vi "Add Menu Items.vi"(7 "Menu control":enum16{"Pulse", "Post-process", "Monitor"}(ring), 8 "error in (no error)":errorcluster, 9 "Reset":bool, 10 "Item Names":string[](array[string]), 11 "Monitor-Pulse in":refnum<class "Monitor-Pulse.lvclass">) -> (0 "error out":errorcluster, 3 "Monitor-Pulse out":refnum<class "Monitor-Pulse.lvclass">)   [LabVIEW 2016, in "Monitor-Pulse.lvclass"]
uses:
  Monitor-Pulse.lvclass
  Monitor-Pulse.lvclass/Monitor-Pulse.ctl
  Controllers/Application Controller/Application Controller.lvclass
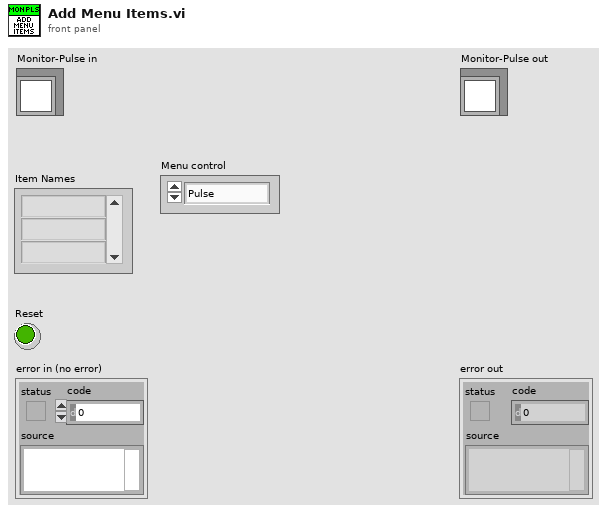
[diagram p1: front panel]
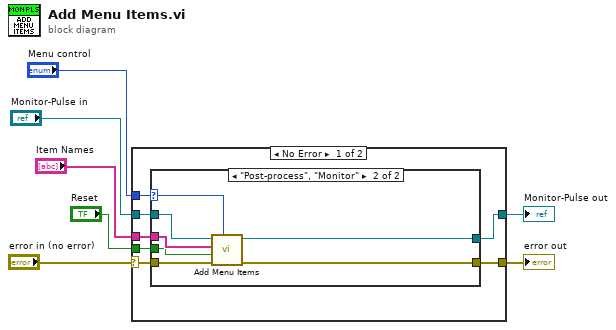
[diagram p0: block diagram]
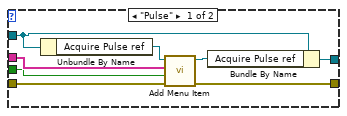
[diagram p2: hidden frame]
diagram:
  n1 = case shown="No Error" "error in (no error)" {
    selector: "error in (no error)" -> [w10 w31]
    tunnel: [w9 w31] -> w6
    tunnel: [w14 w30] -> w4
    tunnel: "Monitor-Pulse in" -> [w11 w30]
    tunnel: "Item Names" -> [w13 _]
    tunnel: "Reset" -> [w12 _]
    tunnel: "Menu control" -> [w8 _]
    frame No Error {
      n2 = case shown="\"Post-process\", \"Monitor\"" w8 {
        selector: w8 -> [_ w23]
        tunnel: [w20 w27] -> w14
        tunnel: w13 -> [w19 w26]
        tunnel: w12 -> [w18 w25]
        tunnel: w11 -> [w17 w29]
        tunnel: w10 -> [w16 w28]
        tunnel: [w15 w24] -> w9
        frame "Pulse" {
          n3 = Unbundle By Name(w17) -> ("Acquire Pulse ref"=w22:refnum<vi>)
          n4 = call "Add Menu Item.vi"("error in (no error)"=w16, "Reset"=w18, "Item Names"=w19, "Queed Listbox ref"=w22) -> ("error out"=w15:errorcluster, "Queed Listbox ref out"=w21:refnum<vi>)  [unwired: 5 in, 1 out]
          n5 = Bundle By Name(cluster=w17, "Acquire Pulse ref"=w21) -> (w20:refnum<class "Monitor-Pulse.lvclass">)
        }
        frame "Post-process", "Monitor" {
          n6 = call-parent "Add Menu Items.vi"("Menu control"=w23, "error in (no error)"=w28, "Reset"=w25, "Item Names"=w26, "Monitor-Pulse in"=w29) -> ("error out"=w24:errorcluster, "Monitor-Pulse out"=w27:refnum<class "Monitor-Pulse.lvclass">)  [unwired: 5 in]
        }
      }
    }
    frame Error {
    }
  }
  "error out" <- w6
  "Monitor-Pulse out" <- w4
